vi "Omron TCP FINS-Response Data.vi"(8 "error in":errorcluster, 11 "Buffer Data In":T1) -> (0 "error out":errorcluster, 2 "Data":i16[](array[numeric]), 3 "Buffer Data Out":T1)   [LabVIEW 2016]
uses:
  Data Def/Omron TCP FINS-Buffer Data.ctl
  Data Def/Omron TCP FINS-Command Code.ctl
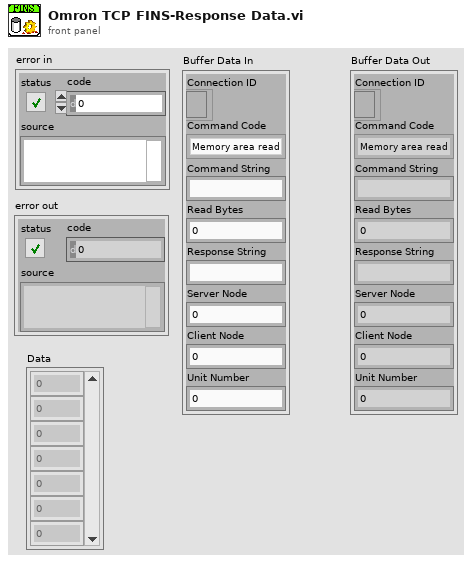
[diagram p1: front panel]
types:
  T1 = typedef "Omron TCP FINS-Buffer Data.ctl" = cluster{"Connection ID":refnum<k5>, "Command Code":T2, "Command String":string, "Read Bytes":i32, "Response String":string, "Server Node":u8, "Client Node":u8, "Unit Number":u8}
  T2 = typedef "Omron TCP FINS-Command Code.ctl" = enum16{"Memory area read", "Memory area write"}
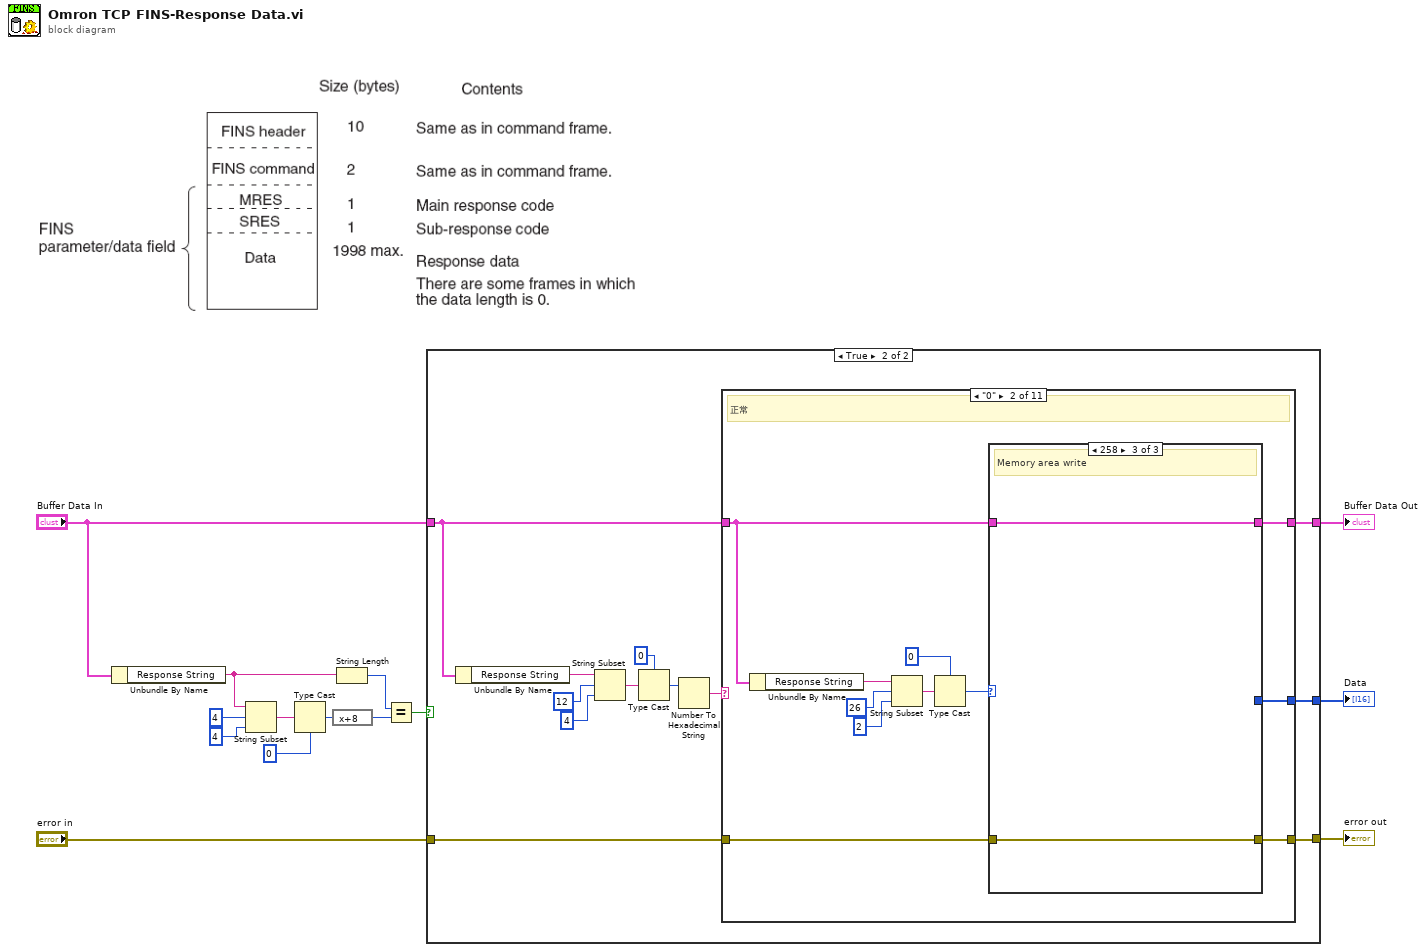
[diagram p0: block diagram]
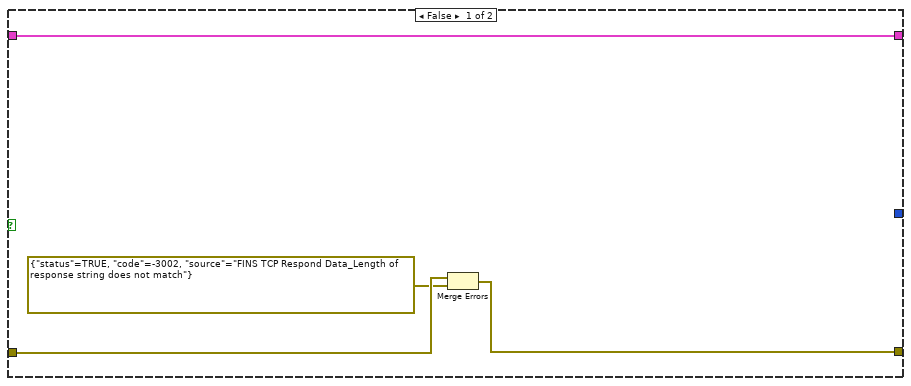
[diagram p2: hidden frame]
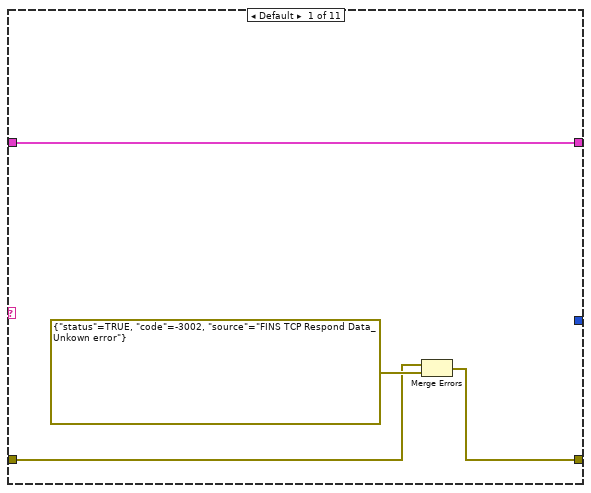
[diagram p3: hidden frame]
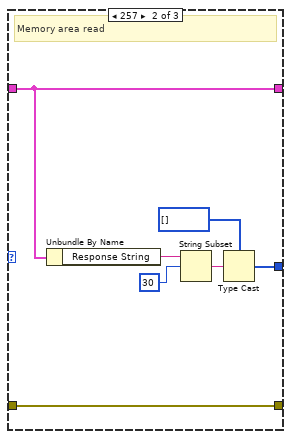
[diagram p5: hidden frame]
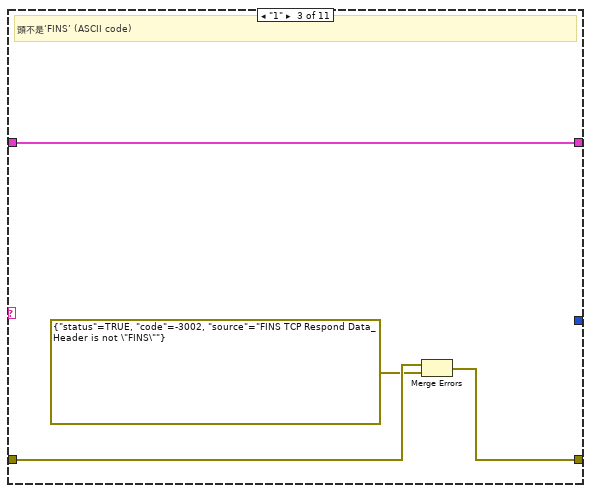
[diagram p6: hidden frame]
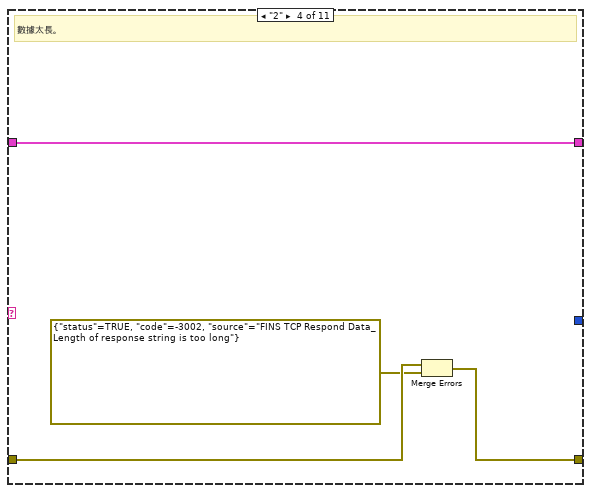
[diagram p7: hidden frame]
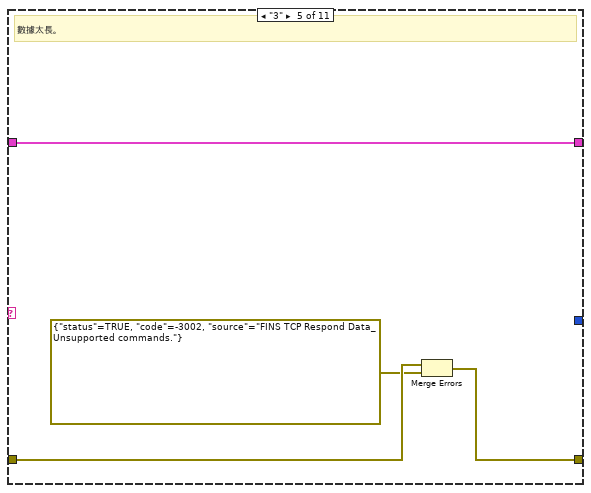
[diagram p8: hidden frame]
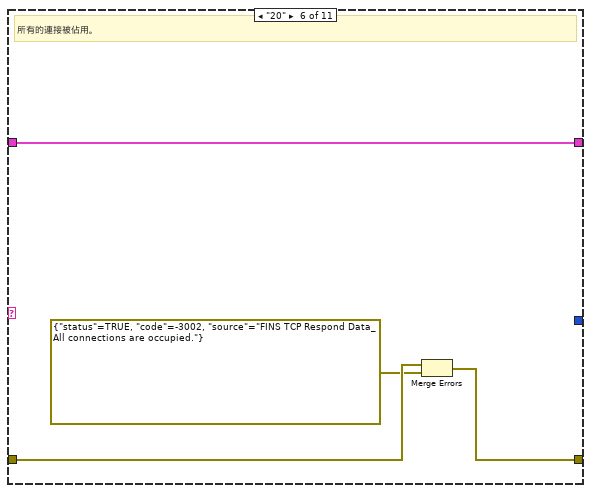
[diagram p9: hidden frame]
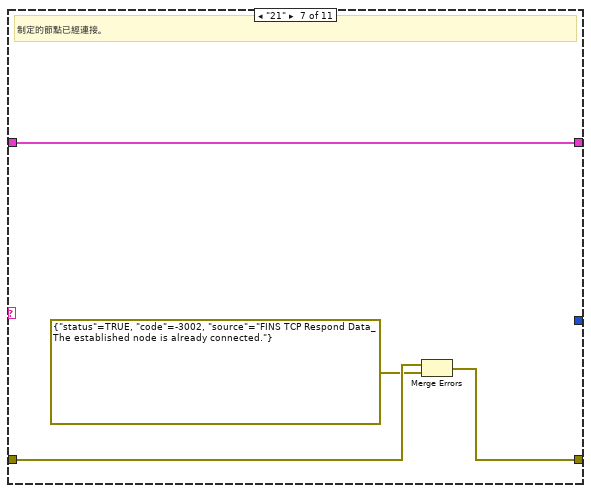
[diagram p10: hidden frame]
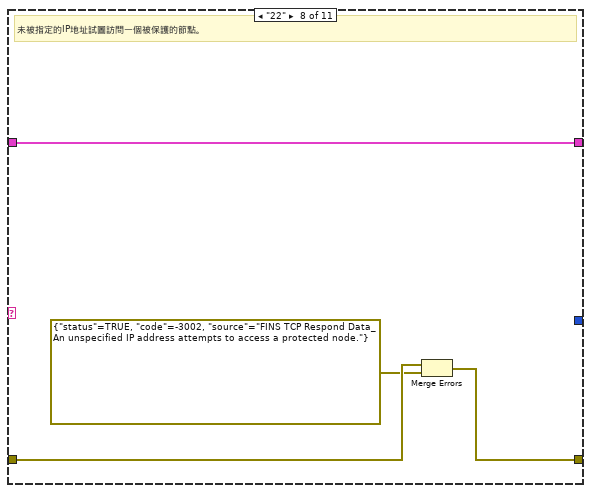
[diagram p11: hidden frame]
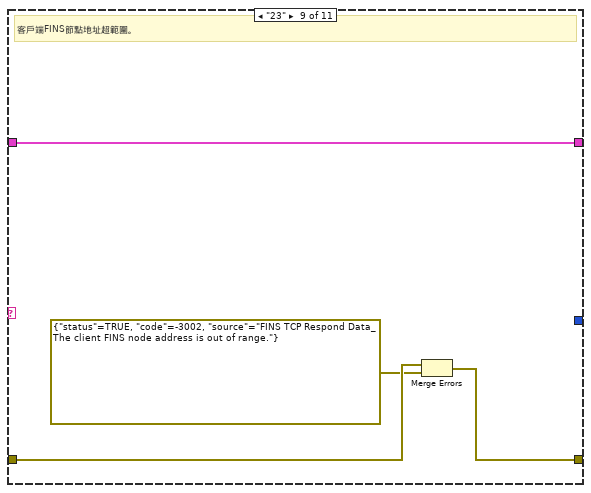
[diagram p12: hidden frame]
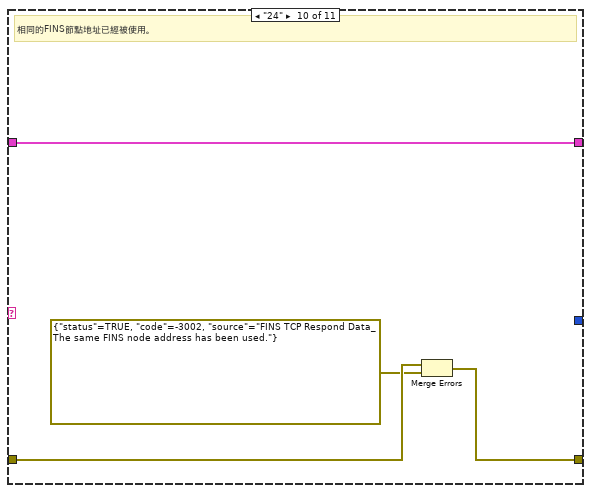
[diagram p13: hidden frame]
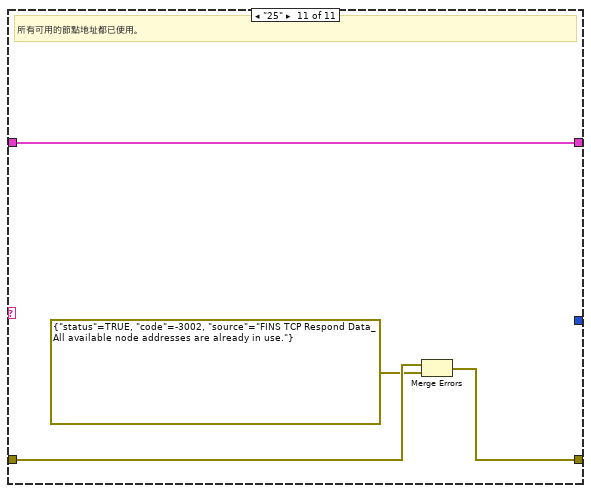
[diagram p14: hidden frame]
diagram:
  n1 = Unbundle By Name("Buffer Data In") -> ("Response String"=w8:string)
  n2 = String Subset(string=w8, offset (0)=4, length (rest)=4 ("length (rest)")) -> (substring=w10:string)
  n3 = Type Cast(type=0, x=w10) -> (*(type *) &x=w7:i32)
  n4 = expression code="x+8"(w7) -> (w6:i32)
  n5 = String Length(string=w8) -> (length=w5:i32)
  n6 = Equal?(x=w5, y=w6) -> (x = y?=w4:bool)
  n7 = case shown="True" w4 {
    tunnel: "error in" -> [w18 w24]
    tunnel: [w17 w22] -> w13
    tunnel: "Buffer Data In" -> [w15 w21]
    tunnel: [_ w20] -> w2
    tunnel: [w15 w19] -> w1
    frame False {
      n8 = Merge Errors(w18, errorcluster {"status"=TRUE, "code"=-3002, "source"="FINS TCP Respond Data_Length of response string does not match"} ("error in")) -> (w17:errorcluster)
    }
    frame True {
      n9 = Unbundle By Name(w21) -> ("Response String"=w30:string)
      n10 = String Subset(string=w30, offset (0)=12, length (rest)=4 ("length (rest)")) -> (substring=w25:string)
      n11 = Type Cast(type=0, x=w25) -> (*(type *) &x=w27:i32)
      n12 = Number To Hexadecimal String(2:w27) -> (0:w23:string)  [unwired: 1 in]
      n13 = case shown="\"0\"" w23 {
        tunnel: w24 -> [w33 w40 w60 w64 w68 w72 w76 w80 w84 w88 w92]
        tunnel: [w32 w38 w58 w62 w66 w70 w74 w78 w82 w86 w90] -> w22
        tunnel: w21 -> [w31 w37 w57 w61 w65 w69 w73 w77 w81 w85 w89]
        tunnel: [_ w36 _ _ _ _ _ _ _ _ _] -> w20
        tunnel: [w31 w35 w57 w61 w65 w69 w73 w77 w81 w85 w89] -> w19
        frame Default {
          n14 = Merge Errors(w33, errorcluster {"status"=TRUE, "code"=-3002, "source"="FINS TCP Respond Data_Unkown error"} ("error in")) -> (w32:errorcluster)
        }
        frame "0" {
          # "正常"
          n15 = Unbundle By Name(w37) -> ("Response String"=w43:string)
          n16 = String Subset(string=w43, offset (0)=26, length (rest)=2 ("length (rest)")) -> (substring=w42:string)
          n17 = Type Cast(type=u16 0, x=w42) -> (*(type *) &x=w39:u16)
          n18 = case shown="258" w39 {
            tunnel: w40 -> [w47 w49 w56]
            tunnel: [w47 w49 w56] -> w38
            tunnel: w37 -> [w46 w48 w55]
            tunnel: [_ w50 _] -> w36
            tunnel: [w46 w48 w55] -> w35
            frame Default {
            }
            frame 257 {
              # "Memory area read"
              n19 = Unbundle By Name(w48) -> ("Response String"=w52:string)
              n20 = String Subset(string=w52, offset (0)=30) -> (substring=w53:string)  [unwired: 1 in]
              n21 = Type Cast(type=i16[] [], x=w53) -> (*(type *) &x=w50:i16[])
            }
            frame 258 {
              # "Memory area write"
            }
          }
        }
        frame "1" {
          # "頭不是‘FINS’ (ASCII code)"
          n22 = Merge Errors(w60, errorcluster {"status"=TRUE, "code"=-3002, "source"="FINS TCP Respond Data_Header is not \"FINS\""} ("error in")) -> (w58:errorcluster)
        }
        frame "2" {
          # "數據太長。"
          n23 = Merge Errors(w64, errorcluster {"status"=TRUE, "code"=-3002, "source"="FINS TCP Respond Data_Length of response string is too long"} ("error in")) -> (w62:errorcluster)
        }
        frame "3" {
          # "數據太長。"
          n24 = Merge Errors(w68, errorcluster {"status"=TRUE, "code"=-3002, "source"="FINS TCP Respond Data_Unsupported commands."} ("error in")) -> (w66:errorcluster)
        }
        frame "20" {
          # "所有的連接被佔用。"
          n25 = Merge Errors(w72, errorcluster {"status"=TRUE, "code"=-3002, "source"="FINS TCP Respond Data_All connections are occupied."} ("error in")) -> (w70:errorcluster)
        }
        frame "21" {
          # "制定的節點已經連接。"
          n26 = Merge Errors(w76, errorcluster {"status"=TRUE, "code"=-3002, "source"="FINS TCP Respond Data_The established node is already connected."} ("error in")) -> (w74:errorcluster)
        }
        frame "22" {
          # "未被指定的IP地址試圖訪問一個被保護的節點。"
          n27 = Merge Errors(w80, errorcluster {"status"=TRUE, "code"=-3002, "source"="FINS TCP Respond Data_An unspecified IP address attempts to access a protected node."} ("error in")) -> (w78:errorcluster)
        }
        frame "23" {
          # "客戶端FINS節點地址超範圍。"
          n28 = Merge Errors(w84, errorcluster {"status"=TRUE, "code"=-3002, "source"="FINS TCP Respond Data_The client FINS node address is out of range."} ("error in")) -> (w82:errorcluster)
        }
        frame "24" {
          # "相同的FINS節點地址已經被使用。"
          n29 = Merge Errors(w88, errorcluster {"status"=TRUE, "code"=-3002, "source"="FINS TCP Respond Data_The same FINS node address has been used."} ("error in")) -> (w86:errorcluster)
        }
        frame "25" {
          # "所有可用的節點地址都已使用。"
          n30 = Merge Errors(w92, errorcluster {"status"=TRUE, "code"=-3002, "source"="FINS TCP Respond Data_All available node addresses are already in use."} ("error in")) -> (w90:errorcluster)
        }
      }
    }
  }
  "error out" <- w13
  "Buffer Data Out" <- w1
  "Data" <- w2
